vi "Read Template Paths.vi"(8 "error in (no error)":errorcluster, 11 "CS++Actor in":refnum<class "CS++Actor.lvclass">) -> (0 "error out":errorcluster, 2 "Template Paths":path[](array[path]), 3 "CS++Actor out":refnum<class "CS++Actor.lvclass">)   [LabVIEW 2014, in "CS++Actor.lvlib" / "CS++Actor.lvclass"]
uses:
  CS++Actor.lvclass
  CS++Actor.lvclass/CS++Actor.ctl
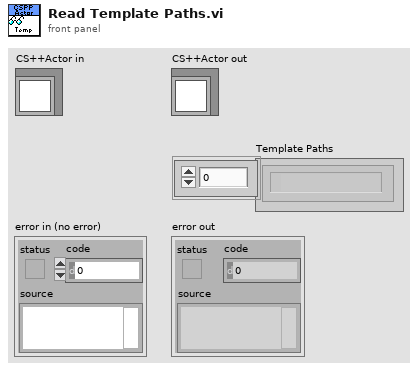
[diagram p1: front panel]
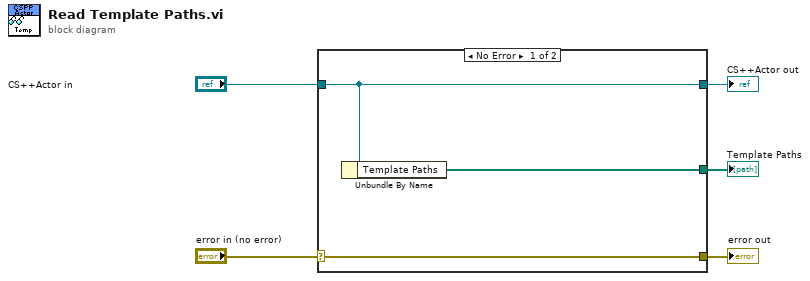
[diagram p0: block diagram]
diagram:
  n1 = case shown="No Error" "error in (no error)" {
    selector: "error in (no error)" -> [w8 w9]
    tunnel: [w8 w9] -> w4
    tunnel: [w7 w10] -> w2
    tunnel: "CS++Actor in" -> [w7 w10]
    tunnel: [w6 _] -> w1
    frame No Error {
      n2 = Unbundle By Name(w7) -> ("Template Paths"=w6:path[])
    }
    frame Error {
    }
  }
  "error out" <- w4
  "CS++Actor out" <- w2
  "Template Paths" <- w1
